vi "Process.vi"(8 "error in":errorcluster, 11 "Logger.Error":refnum<class "Logger.Error.lvclass">) -> (0 "error out":errorcluster, 3 "Logger.Error out":refnum<class "Logger.Error.lvclass">)   [LabVIEW 2019, in "Logger.Error.lvlib" / "Logger.Error.lvclass"]
doc: "---------------------------------------------------------------\nJKI State Machine Objects™\nhttp://jki.net/state-machine-objects/\nCopyright (C) 2005-2015, JKI <info@jki.net>\nALL RIGHTS RESERVED"
uses:
  Logger.Error.lvclass
  C:/Program Files (x86)/National Instruments/LabVIEW 2019/vi.lib/JKI/JKI SMO/smo.lvlibp/SMO/SMO.lvclass
  Logger.Error.lvclass/Logger.Error.ctl
  <vilib>/Utility/file.llb/Write Delimited Spreadsheet (string).vi
  <userlib>/LevyLab/Logger/Logger/Logger.lvclass
  <vilib>/JKI/JKI SMO/smo.lvlibp/SMO/SMO.lvclass
  <userlib>/LevyLab/Debug/Debug.lvlib
panel:
  out "Status":string
  out "State History":string
  # "error Logger"
  # "For instructions on how to use the JKI State Machine Objects, examples and video tutorials, visit:\nhttp://jki.net/state-machine-objects/\n\nJKI State Machine Objects™\nhttp://jki.net/state-machine-objects/\nCopyright (C) 2005-2015, JKI <info@jki.net>\nALL RIGHTS RESERVED"
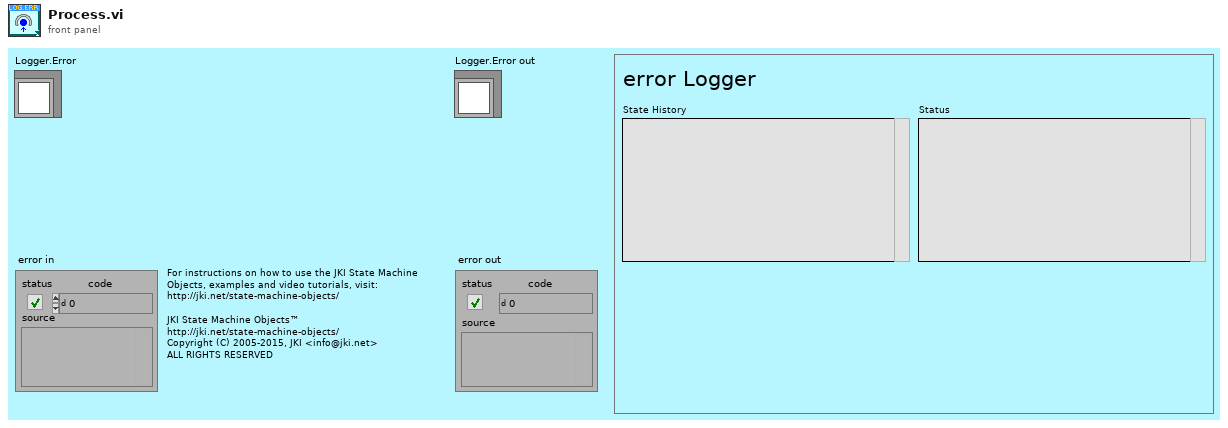
[diagram p1: front panel]
types:
  T1 = enum32{"invalid app kind", "Development System", "Run Time System", "Student Edition", "Embedded LabVIEW", "Evaluation", "Custom"}
  T2 = enum32{"Invalid", "Standard", "Closed", "Hidden", "Minimized", "Maximized"}
  T3 = cluster{"Core":cluster{"Current VI Reference":refnum<vi>, "Close Panel on Exit?":bool, "Last Error":cluster{"error":errorcluster, "previous state":string, "remaining states":string}, "Shutdown?":bool}, "SelfRef":refnum<class "Logger.Error.lvclass">, "path":path, "SMOs":refnum<class "SMO.lvclass">[], "error to log":errorcluster}
  T4 = cluster{"Current VI Reference":refnum<vi>, "Close Panel on Exit?":bool, "Last Error":cluster{"error":errorcluster, "previous state":string, "remaining states":string}, "Shutdown?":bool}
  T5 = typedef "Debug.lvlib/Attribute.Debug.lvclass/DebugBehavior.ctl" = enum16{"Normal", "Debug"}
  T6 = typedef "smo.lvlibp/SMO.lvclass/Protected Events.ctl" = cluster{"StopProcesses":refnum<user-event>, "AbortProcesses":refnum<user-event>, "Config Changed":refnum<user-event>, "Dependency":refnum<user-event>}
  T7 = typedef "smo.lvlibp/SMO.lvclass/Public Events.ctl" = cluster{"Error":refnum<user-event>, "State":refnum<user-event>, "Reserve State":refnum<user-event>}
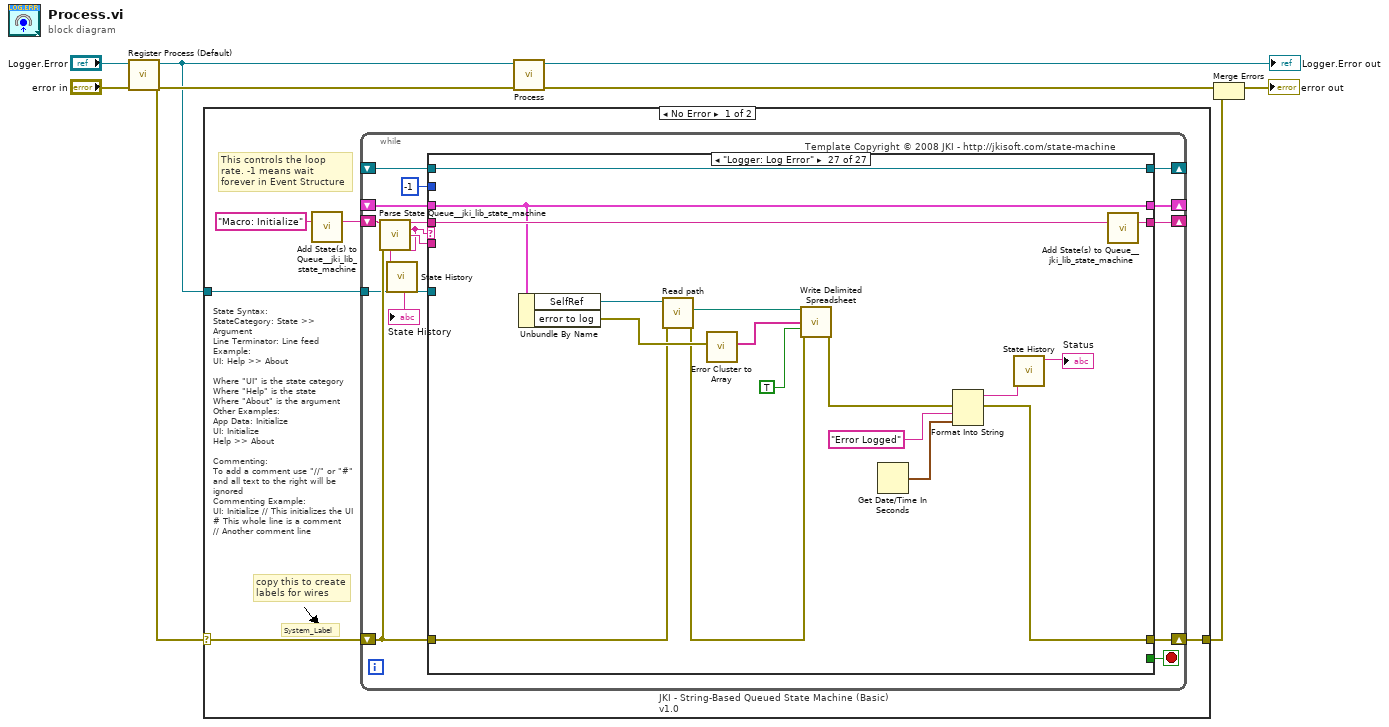
[diagram p0: block diagram]
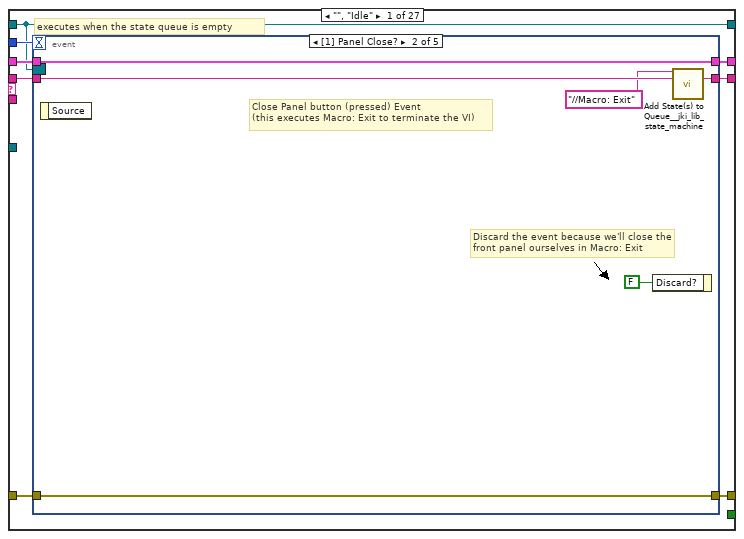
[diagram p2: hidden frame]
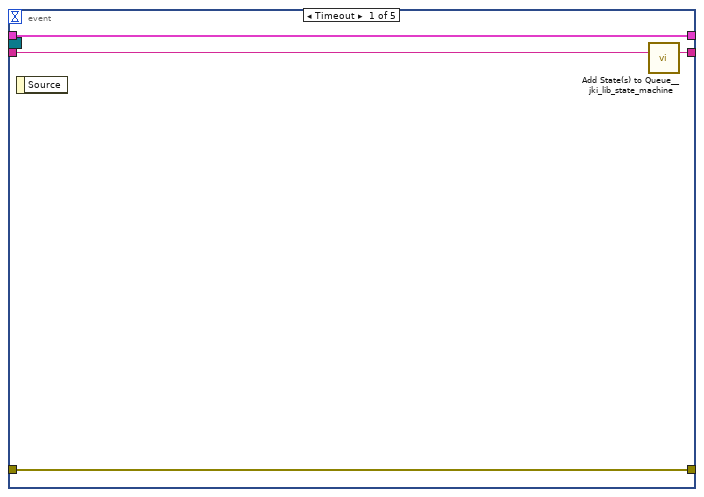
[diagram p3: hidden frame]
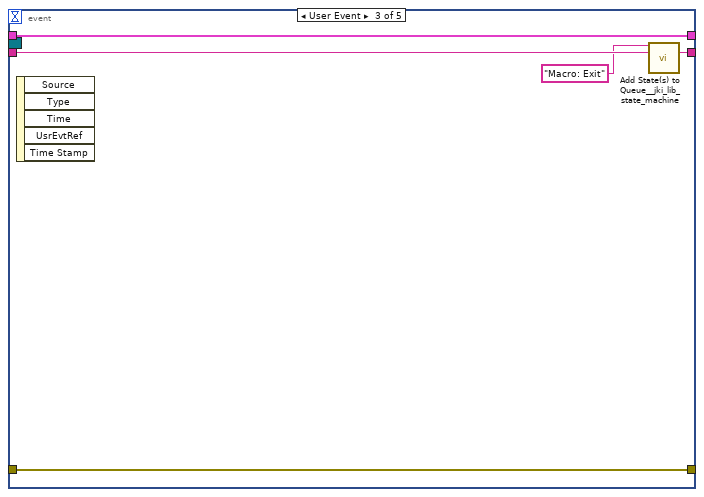
[diagram p4: hidden frame]
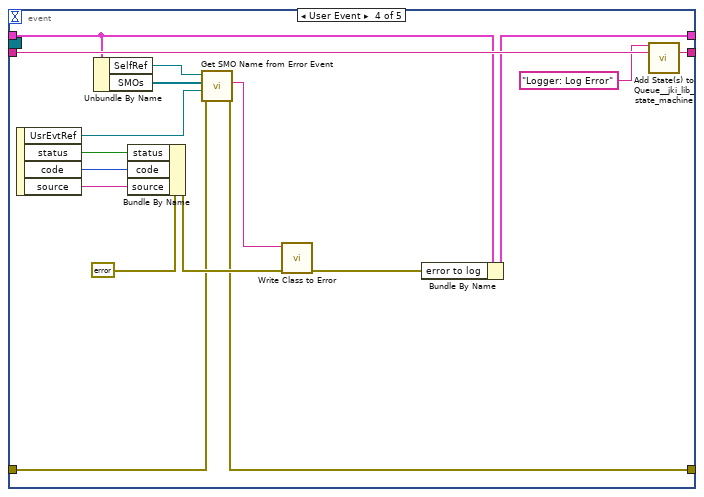
[diagram p5: hidden frame]
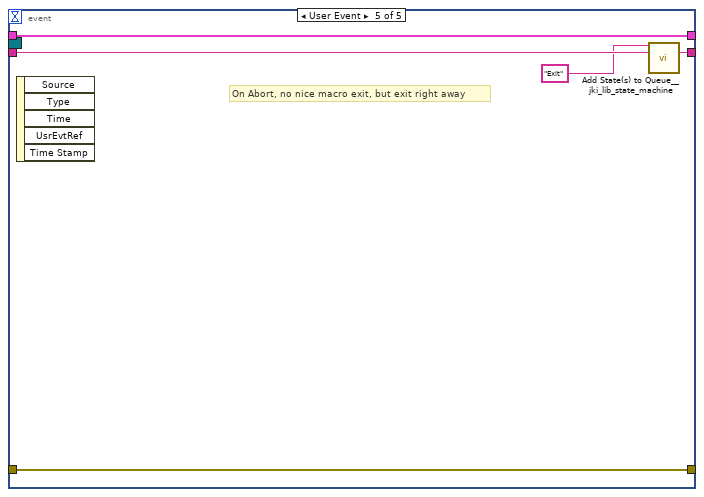
[diagram p6: hidden frame]
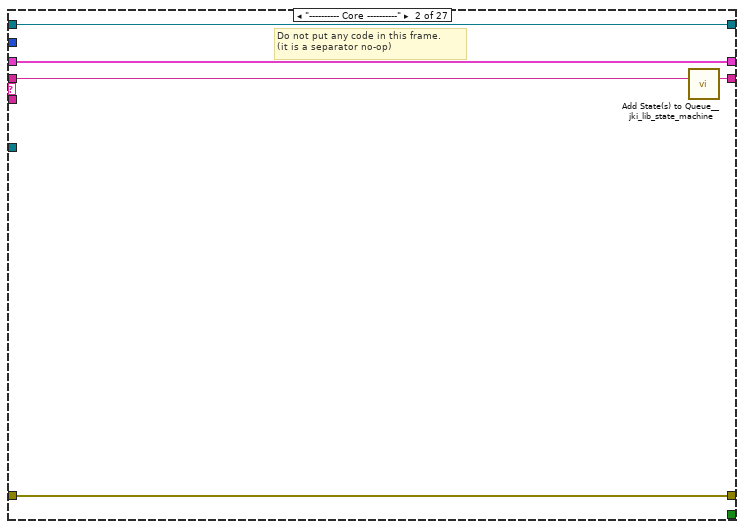
[diagram p7: hidden frame]
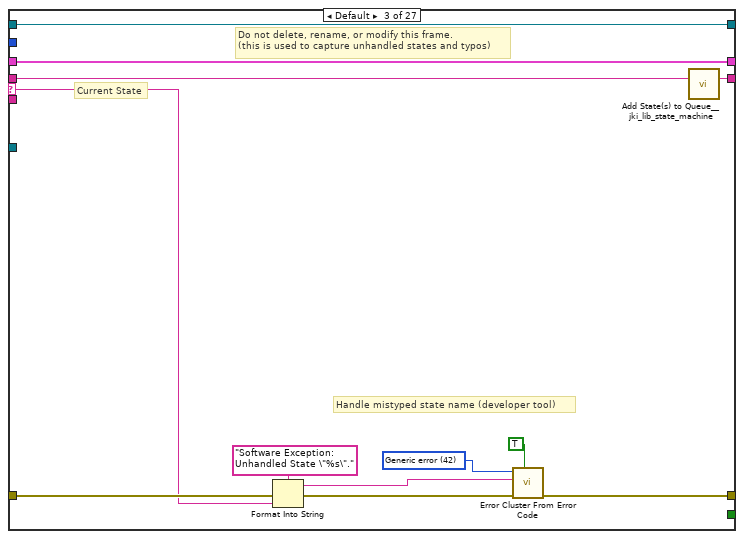
[diagram p8: hidden frame]
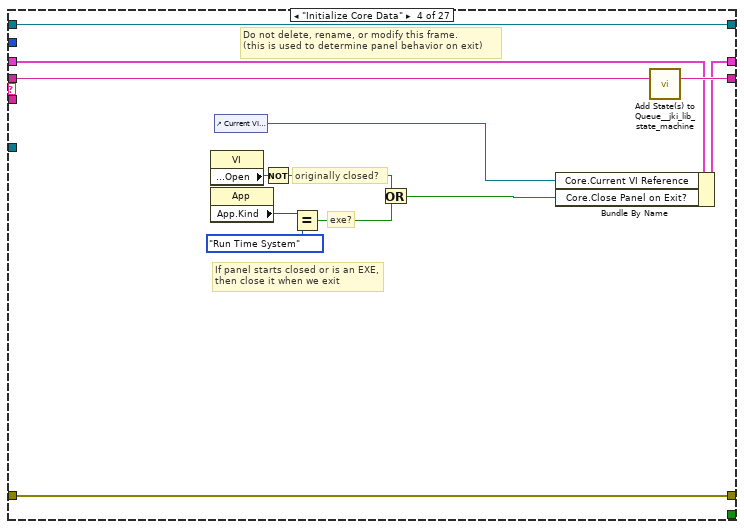
[diagram p9: hidden frame]
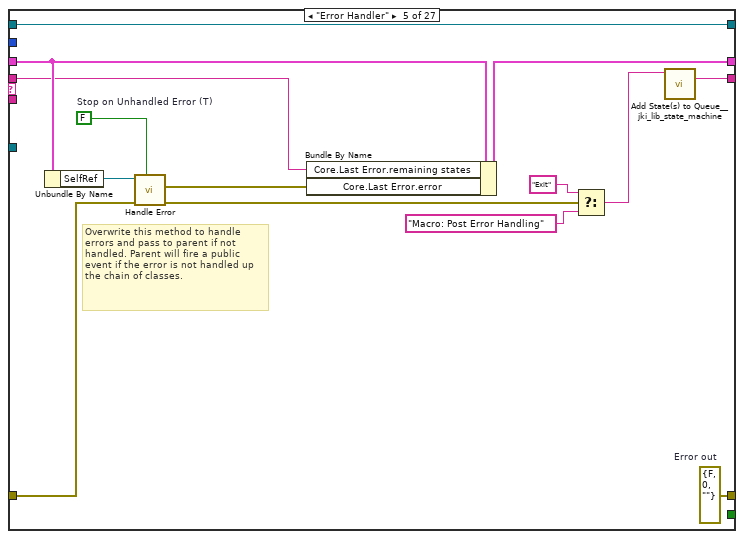
[diagram p10: hidden frame]
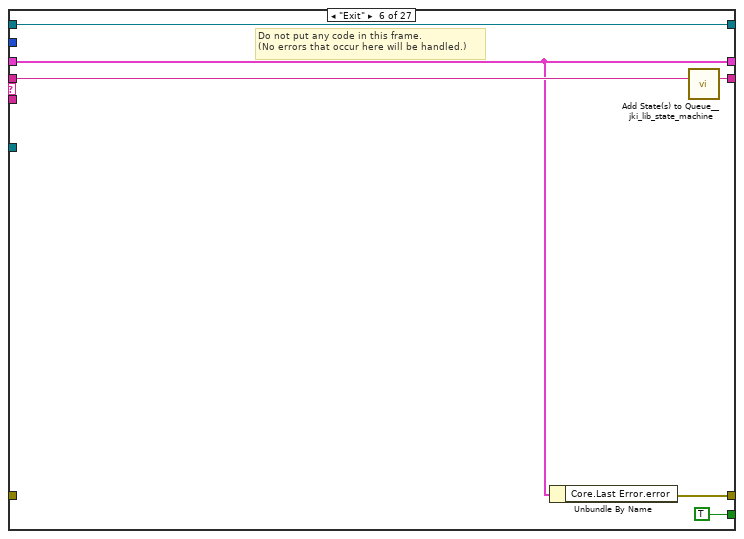
[diagram p11: hidden frame]
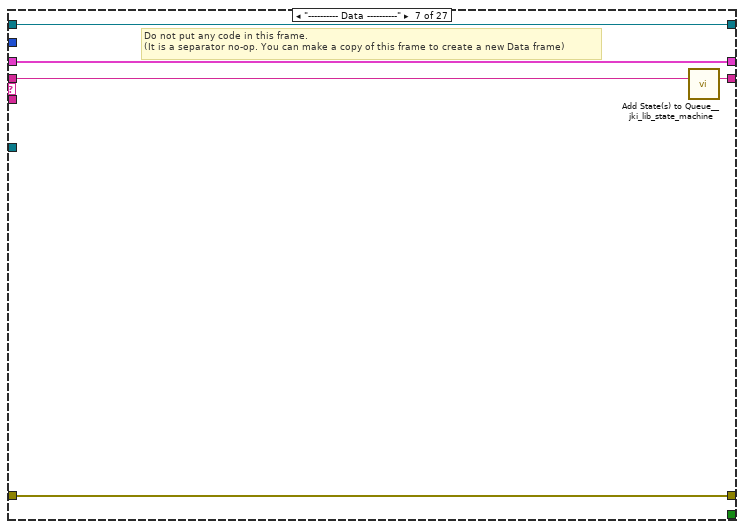
[diagram p12: hidden frame]
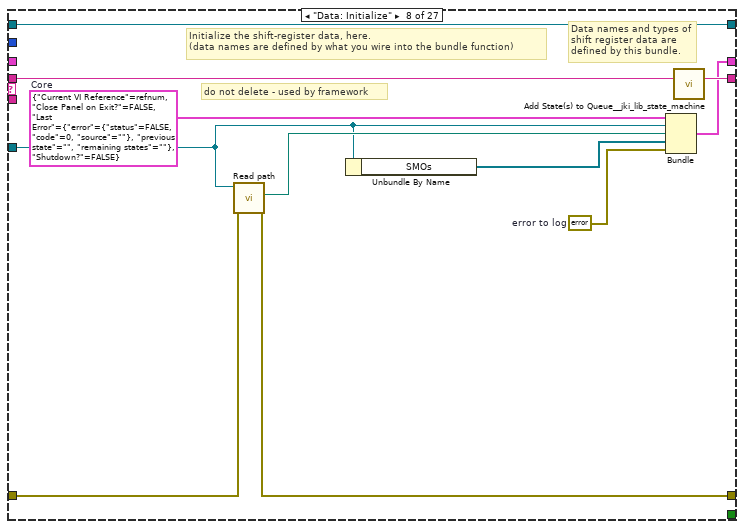
[diagram p13: hidden frame]
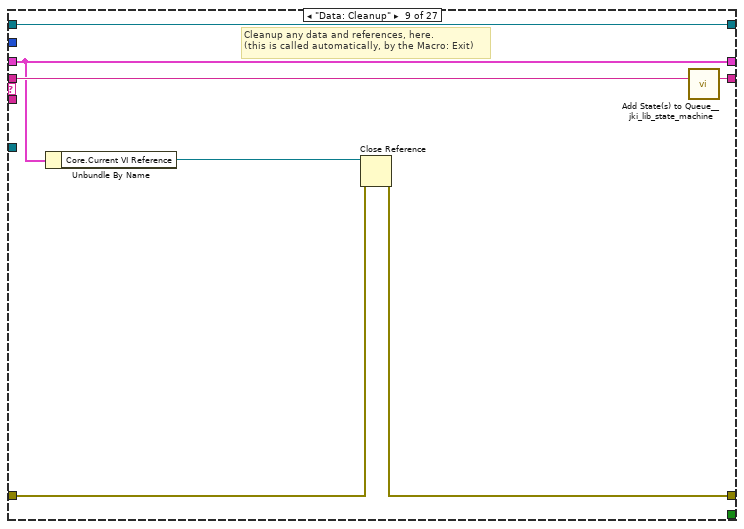
[diagram p14: hidden frame]
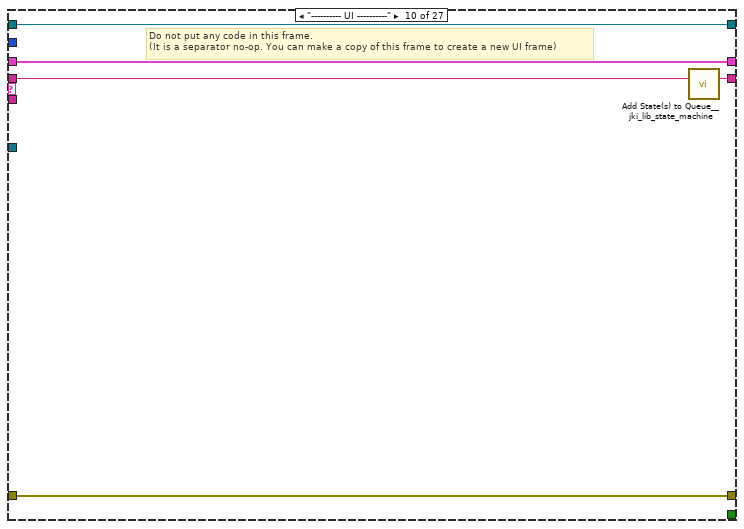
[diagram p15: hidden frame]
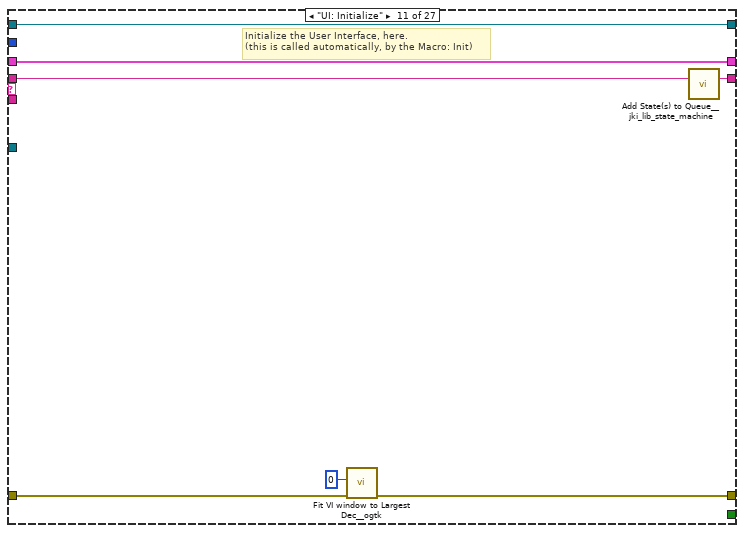
[diagram p16: hidden frame]
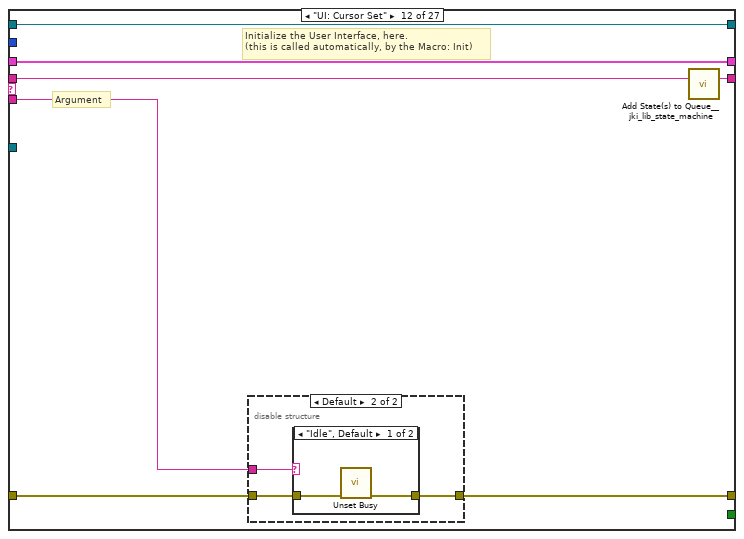
[diagram p17: hidden frame]
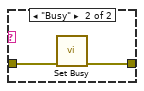
[diagram p19: hidden frame]
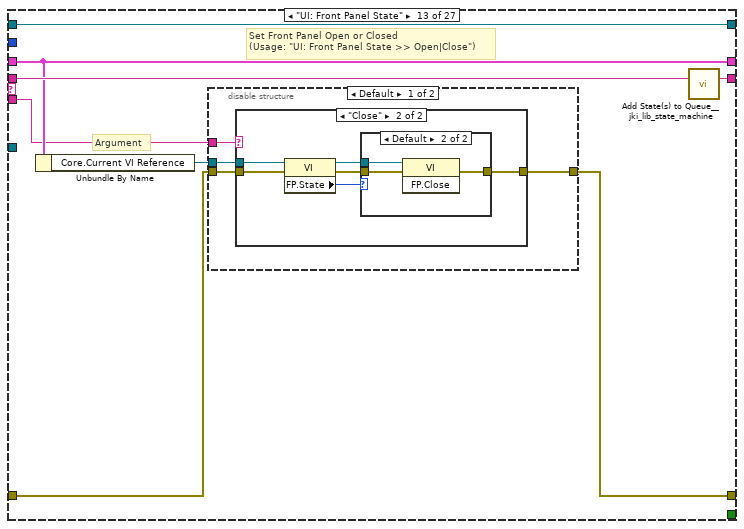
[diagram p20: hidden frame]
diagram:
  n1 = call <vilib>:"Register Process (Default).vi"("error in (no error)"="error in", "SMO"="Logger.Error") -> ("error out"=w5:errorcluster, "SelfRef"=w4:refnum<class "Logger.Error.lvclass">)  [unwired: 8 in]
  n2 = case shown="No Error" w5 {
    selector: w5 -> [w10 w365]
    tunnel: w4 -> [w11 _]
    tunnel: [w9 w365] -> w1
    frame No Error {
      # "State Syntax:\nStateCategory: State >> Argument\nLine Terminator: Line feed\nExample:\nUI: Help >> About\n\nWhere \"UI\" is the state category\nWhere \"Help\" is the state\nWhere \"About\" is the argument\nOther Examples:\nApp Data: Initialize\nUI: Initialize\nHelp >> About\n\nCommenting:\nTo add a comment use \"//\" or \"#\" and all text to the right will be ignored\nCommenting Example:\nUI: Initialize // This initializes the UI\n# This whole line is a comment\n// Another comment line"
      # "copy this to create labels for wires"
      # "This controls the loop rate. -1 means wait forever in Event Structure"
      # "System_Label"
      n3 = call <vilib>:"Add State(s) to Queue__jki_lib_state_machine.vi"("State(s) in (\"\")"="Macro: Initialize") -> ("States Out"=w13:string)  [unwired: 14 in]
      n4 = while "JKI - String-Based Queued State Machine (Basic) v1.0" {
        shift-right: [w22] -> _
        shift-left: _ -> [w14]
        shift-right: [w25] -> w9
        shift-left: w10 -> [w20]
        shift-right: [w24] -> _
        shift-left: w13 -> [w26]
        tunnel: w11 -> [w19]
        shift-right: [w18] -> _
        shift-left: _ -> [w17]
        stop <- w23 stop-if-true
        # "Template Copyright © 2008 JKI - http://jkisoft.com/state-machine"
        n5 = call <vilib>:"Parse State Queue__jki_lib_state_machine.vi"("State Queue"=w26, "Error In (no error)"=w20) -> ("Remaining States"=w28:string, "Current State"=w15:string, "Arguments"=w27:string)  [unwired: 11 in]
        n6 = call <userlib>:"State History.vi"("Current State"=w15) -> ("History"=→"State History":string)  [unwired: 10 in]
        n7 = case shown="\"Logger: Log Error\"" w15 {
          selector: w15 -> [_ _ w80 _ _ _ _ _ _ _ _ _ _ _ _ _ _ _ _ _ _ _ _ _ _ _ _]
          tunnel: w28 -> [w36 w78 w84 w103 w106 w123 w128 w139 w146 w151 w158 w165 w181 w213 w224 w239 w256 w277 w282 w293 w298 w315 w326 w331 w340 w347 w364]
          tunnel: w27 -> [_ _ _ _ _ _ _ _ _ _ _ w159 w175 _ _ _ _ _ _ _ _ _ _ _ _ _ _]
          tunnel: [w33 w76 w86 w100 w113 w118 w126 w131 w142 w149 w153 w160 w178 w211 w215 w226 w254 w275 w280 w284 w296 w311 w322 w327 w336 w341 w349] -> w25
          tunnel: w20 -> [w32 w76 w85 w100 w114 _ w126 w132 w143 w149 w152 w161 w179 w211 w215 w225 w254 w275 w280 w285 w296 w302 w322 w327 w337 w342 w354]
          tunnel: [w35 w77 w83 w102 w117 w122 w127 w138 w145 w150 w157 w164 w180 w212 w223 w238 w255 w276 w281 w292 w297 w314 w325 w330 w339 w346 w363] -> w24
          tunnel: [_ _ _ _ _ TRUE _ _ _ _ _ _ _ _ _ _ _ _ _ _ _ _ _ _ _ _ _] -> w23
          tunnel: [w31 w75 w82 w101 w111 w119 w125 w137 w141 w148 w156 w163 w177 w210 w217 w229 w246 w262 w279 w290 w295 w305 w324 w329 w333 w344 w361] -> w22
          tunnel: -1 ("Timeout") -> [w30 _ _ _ _ _ _ _ _ _ _ _ _ _ _ _ _ _ _ _ _ _ _ _ _ _ _]
          tunnel: w19 -> [_ _ _ _ _ _ _ w130 _ _ _ _ _ _ _ _ _ _ _ _ _ _ _ _ _ _ _]
          tunnel: [w29 w74 w79 w91 w116 w120 w124 w136 w140 w147 w155 w162 w174 w209 w222 w237 w253 w270 w278 w291 w294 w313 w323 w328 w338 w345 w362] -> w18
          tunnel: w17 -> [w29 w74 w79 w91 w116 w120 w124 w136 w140 w147 w155 w162 w174 w209 w222 w237 w253 w270 w278 w291 w294 _ w323 w328 w338 w345 w362]
          tunnel: w14 -> [w34 w75 w82 w94 w112 w119 w125 _ w141 w148 w156 w163 w177 w210 w217 w228 w245 w261 w279 w290 w295 w306 w324 w329 w332 w344 w361]
          frame "", "Idle" {
            # "executes when the state queue is empty"
            n8 = event shown="[1] Panel Close?" {
              selector: w29 -> [_ _ _ _ _]
              dyn-events: _ -> [_ _ _ _ _]
              timeout: w30 -> [_ _ _ _ _]
              tunnel: w36 -> [w40 w46 w51 w68 w73]
              tunnel: [w39 w45 w50 w67 w72] -> w35
              tunnel: w34 -> [w38 w43 w48 w55 w70]
              tunnel: [w37 w44 w49 w57 w71] -> w33
              tunnel: w32 -> [w37 w44 w49 w58 w71]
              tunnel: [w38 w43 w48 w56 w70] -> w31
              event Timeout {
                n9 = event-data() -> ()  [unwired: 1 in, 1 out]
                n10 = call <vilib>:"Add State(s) to Queue__jki_lib_state_machine.vi"("State(s) in (\"\")"=w40) -> ("States Out"=w39:string)  [unwired: 14 in]
              }
              event Panel Close? {
                # "Discard the event because we'll close the front panel ourselves in Macro: Exit"
                # "Close Panel button (pressed) Event\n(this executes Macro: Exit to terminate the VI)"
                n11 = event-data() -> ()  [unwired: 1 in, 1 out]
                n12 = event-data("Discard?"=FALSE) -> ()  [unwired: 1 in, 1 out]
                n13 = call <vilib>:"Add State(s) to Queue__jki_lib_state_machine.vi"("State(s) in Front (\"\")"="//Macro: Exit", "State(s) in (\"\")"=w46) -> ("States Out"=w45:string)  [unwired: 13 in]
              }
              event User Event {
                n14 = event-data() -> ()  [unwired: 1 in, 5 out]
                n15 = call <vilib>:"Add State(s) to Queue__jki_lib_state_machine.vi"("State(s) in Front (\"\")"="Macro: Exit", "State(s) in (\"\")"=w51) -> ("States Out"=w50:string)  [unwired: 13 in]
              }
              event User Event {
                n16 = event-data() -> ("UsrEvtRef"=w62:refnum<user-event>, "status"=w66:bool, "code"=w65:i32, "source"=w64:string)  [unwired: 1 in]
                n17 = Unbundle By Name(w55) -> ("SelfRef"=w52:refnum<class "Logger.Error.lvclass">, "SMOs"=w63:refnum<class "SMO.lvclass">[])
                n18 = Bundle By Name(cluster=errorcluster {"status"=FALSE, "code"=0, "source"=""} ("error in (no error)"), "status"=w66, "code"=w65, "source"=w64) -> (w60:errorcluster)
                n19 = call "Get SMO Name from Error Event.vi"("error in (no error)"=w58, "Error"=w62, "SMOs"=w63, "Logger.Error"=w52) -> ("error out"=w57:errorcluster, "class:SMO name"=w61:string)  [unwired: 5 in, 1 out]
                n20 = call "Write Class to Error.vi"("Error in"=w60, "Calling Class"=w61) -> ("Error out"=w54:errorcluster)  [unwired: 9 in]
                n21 = Bundle By Name(cluster=w55, "error to log"=w54) -> (w56:T3)
                n22 = call <vilib>:"Add State(s) to Queue__jki_lib_state_machine.vi"("State(s) in Front (\"\")"="Logger: Log Error" ("State(s) in Front (\"\")"), "State(s) in (\"\")"=w68) -> ("States Out"=w67:string)  [unwired: 13 in]
              }
              event User Event {
                # "On Abort, no nice macro exit, but exit right away"
                n23 = event-data() -> ()  [unwired: 1 in, 5 out]
                n24 = call <vilib>:"Add State(s) to Queue__jki_lib_state_machine.vi"("State(s) in Front (\"\")"="Exit", "State(s) in (\"\")"=w73) -> ("States Out"=w72:string)  [unwired: 13 in]
              }
            }
          }
          frame "---------- Core ----------" {
            # "Do not put any code in this frame.\n(it is a separator no-op)"
            n25 = call <vilib>:"Add State(s) to Queue__jki_lib_state_machine.vi"("State(s) in (\"\")"=w78) -> ("States Out"=w77:string)  [unwired: 14 in]
          }
          frame Default {
            w89 = 42 items=["No error", "Argument error", "Memory is full", "Out of zone", "End of file", "File already open", "Generic file I/O error", "File not found", "File permission error", "Disk is full", "Duplicate path", "Too many files open", "System feature not enabled", "Resource file not found", "Cannot add resource", "Resource not found", "Image not found", "Image memory error", "Pen does not exist", "Config type invalid", "Config token not found", "Config parse error", "Config memory error", "Bad external code format", "Bad external code offset", "External code not present", "Null window", "Destroy window error", "Null menu", "Print aborted", "Bad print record", "Print driver error", "Windows error during printing", "Memory error during printing", "Print dialog error", "Generic print error", "Invalid device refnum", "Device not found", "Device parameter error", "Device unit error", "Cannot open device", "Device call aborted", "Generic error", "Cancelled by user", "Object ID too low", "Object ID too high", "Object not in heap", "Unknown heap", "Unknown object (invalid DefProc)", "Unknown object (DefProc not in table)", "Message out of range", "Invalid (null) method", "Unknown message", "Manager call not supported", "Bad address", "Network operation in progress", "Network operation timed out", "Connection is busy", "Network attribute not supported", "Network error", "Address in use", "System out of memory", "Connection aborted", "Connection refused", "Not connected", "Already connected", "Connection closed", "Initialization error (interapplication manager)", "Bad occurrence", "Wait on unbound occurrence handler", "Occurrence queue overflow", "Datalog type conflict", "Unused", "Unrecognized type (interapplication manager)", "Memory corrupt", "Failed to make temporary DLL", "Old CIN version", "Drag socket not found", "Failed to load drop-object", "Failed to register OLE object", "Failed to release OLE object", "Format specifier type mismatch", "Unknown format specifier", "Too few format specifiers", "Too many format specifiers", "Scan failed", "Newer CIN version", "Error converting to variant", "Runtime menu error", "Password tampered", "Variant attribute not found", "Incompatible variant data type", "Event data is not available", "Event Store is not present", "Occurrence is not found", "Event Queue is not created", "Event info is not available", "Refnum passed is NULL", "Error retrieving Class GUID", "Error retrieving CoClass GUID", "Error retrieving TypeLib GUID.", "Bad built application magic bytes.", "Specific driver is different from the specific driver associated with the Logical Name.", "There is no session opened to the class driver.", "Max Error", "MAX - Error with config objects", "MAX - Error loading configuration", "MAX - Group not supported"]
            # "Current State"
            # "Do not delete, rename, or modify this frame.\n(this is used to capture unhandled states and typos)"
            # "Handle mistyped state name (developer tool)"
            n26 = Format Into String(format string="Software Exception: Unhandled State \"%s\"." ("message"), error in=w85, w80) -> (resulting string=w88:string, error out=w87:errorcluster)  [unwired: 1 in]
            n27 = call <vilib>:"Error Cluster From Error Code.vi"("show call chain? (False)"=TRUE, "error in (no error)"=w87, "error message (\"\")"=w88, "error code (0)"=w89) -> ("error out"=w86:errorcluster)  [unwired: 5 in]
            n28 = call <vilib>:"Add State(s) to Queue__jki_lib_state_machine.vi"("State(s) in (\"\")"=w84) -> ("States Out"=w83:string)  [unwired: 14 in]
          }
          frame "Initialize Core Data" {
            # "Do not delete, rename, or modify this frame.\n(this is used to determine panel behavior on exit)"
            # "originally closed?"
            # "exe?"
            # "If panel starts closed or is an EXE, then close it when we exit"
            n29 = property class="VI"() -> ("Front Panel.Open"=w99:bool)  [unwired: 2 in, 2 out]
            n30 = property class="App"() -> ("App.Kind"=w98:T1)  [unwired: 2 in, 2 out]
            n31 = control-ref of="Current VI Reference"() -> (w92:refnum<vi>)
            n32 = Not(x=w99) -> (.not. x?=w96:bool)
            n33 = Equal?(x=w98, y=T1."Run Time System" ("Application:Kind")) -> (x = y?=w95:bool)
            n34 = Or(x=w96, y=w95) -> (x .or. y?=w93:bool)
            n35 = Bundle By Name(cluster=w94, "Core.Current VI Reference"=w92, "Core.Close Panel on Exit?"=w93) -> (w101:T3)
            n36 = call <vilib>:"Add State(s) to Queue__jki_lib_state_machine.vi"("State(s) in (\"\")"=w103) -> ("States Out"=w102:string)  [unwired: 14 in]
          }
          frame "Error Handler" {
            w107 = FALSE  # Stop on Unhandled Error (T)
            w113 = errorcluster {"status"=FALSE, "code"=0, "source"=""}  # Error out
            # "Overwrite this method to handle errors and pass to parent if not handled. Parent will fire a public event if the error is not handled up the chain of classes."
            n37 = Unbundle By Name(w112) -> ("SelfRef"=w115:refnum<class "Logger.Error.lvclass">)
            n38 = call-dynamic "Handle Error.vi"("Stop on Unhandled Error (T)"=w107, "error in"=w114, "SMO"=w115) -> ("handling error"=w108:errorcluster, "Unhandled error"=w104:errorcluster)  [unwired: 6 in, 1 out]
            n39 = Bundle By Name(cluster=w112, "Core.Last Error.remaining states"=w106, "Core.Last Error.error"=w104) -> (w111:T3)
            n40 = Select(t="Exit", s=w108, f="Macro: Post Error Handling") -> (s? t:f=w110:string)
            n41 = call <vilib>:"Add State(s) to Queue__jki_lib_state_machine.vi"("State(s) in Front (\"\")"=w110) -> ("States Out"=w117:string)  [unwired: 14 in]
          }
          frame "Exit" {
            # "Do not put any code in this frame.\n(No errors that occur here will be handled.)"
            n42 = Unbundle By Name(w119) -> ("Core.Last Error.error"=w118:errorcluster)
            n43 = call <vilib>:"Add State(s) to Queue__jki_lib_state_machine.vi"("State(s) in (\"\")"=w123) -> ("States Out"=w122:string)  [unwired: 14 in]
          }
          frame "---------- Data ----------" {
            # "Do not put any code in this frame.\n(It is a separator no-op. You can make a copy of this frame to create a new Data frame)"
            n44 = call <vilib>:"Add State(s) to Queue__jki_lib_state_machine.vi"("State(s) in (\"\")"=w128) -> ("States Out"=w127:string)  [unwired: 14 in]
          }
          frame "Data: Initialize" {
            w133 = errorcluster {"status"=FALSE, "code"=0, "source"=""}  # error to log
            w135 = T4 {"Current VI Reference"=refnum, "Close Panel on Exit?"=FALSE, "Last Error"={"error"={"status"=FALSE, "code"=0, "source"=""}, "previous state"="", "remaining states"=""}, "Shutdown?"=FALSE}  # Core
            # "do not delete - used by framework"
            # "Data names and types of shift register data are defined by this bundle."
            # "Initialize the shift-register data, here.\n(data names are defined by what you wire into the bundle function)"
            n45 = call-dynamic "Read path.vi"("error in (no error)"=w132, "Logger in"=w130) -> ("error out"=w131:errorcluster, "path"=w134:path)  [unwired: 7 in, 1 out]
            n46 = Unbundle By Name(w130) -> ("SMOs"=w129:refnum<class "SMO.lvclass">[])
            n47 = Bundle("Core"=w135, "SelfRef"=w130, "path"=w134, "SMOs"=w129, "error to log"=w133) -> (w137:T3)  [unwired: 1 in]
            n48 = call <vilib>:"Add State(s) to Queue__jki_lib_state_machine.vi"("State(s) in (\"\")"=w139) -> ("States Out"=w138:string)  [unwired: 14 in]
          }
          frame "Data: Cleanup" {
            # "Cleanup any data and references, here.\n(this is called automatically, by the Macro: Exit)"
            n49 = Unbundle By Name(w141) -> ("Core.Current VI Reference"=w144:refnum<vi>)
            n50 = Close Reference(reference=w144, error in (no error)=w143) -> (error out=w142:errorcluster)
            n51 = call <vilib>:"Add State(s) to Queue__jki_lib_state_machine.vi"("State(s) in (\"\")"=w146) -> ("States Out"=w145:string)  [unwired: 14 in]
          }
          frame "---------- UI ----------" {
            # "Do not put any code in this frame.\n(It is a separator no-op. You can make a copy of this frame to create a new UI frame)"
            n52 = call <vilib>:"Add State(s) to Queue__jki_lib_state_machine.vi"("State(s) in (\"\")"=w151) -> ("States Out"=w150:string)  [unwired: 14 in]
          }
          frame "UI: Initialize" {
            # "Initialize the User Interface, here.\n(this is called automatically, by the Macro: Init)"
            n53 = call <userlib>:"Fit VI window to Largest Dec__ogtk.vi"("error in (no error)"=w152, "border spacing (2 px)"=0) -> ("error out"=w153:errorcluster)  [unwired: 4 in, 1 out]
            n54 = call <vilib>:"Add State(s) to Queue__jki_lib_state_machine.vi"("State(s) in (\"\")"=w158) -> ("States Out"=w157:string)  [unwired: 14 in]
          }
          frame "UI: Cursor Set" {
            # "Argument"
            # "Initialize the User Interface, here.\n(this is called automatically, by the Macro: Init)"
            n55 = disable-structure shown="Default" {
              disable-tunnel: w161 -> [w166 w169]
              disable-tunnel: [w166 w168] -> w160
              disable-tunnel: w159 -> [_ w167]
              frame condition #0 {
              }
              frame condition #1 (active) {
                n56 = case shown="\"Idle\", Default" w167 {
                  tunnel: w169 -> [w171 w173]
                  tunnel: [w170 w172] -> w168
                  frame "Idle", Default {
                    n57 = call <vilib>:"Unset Busy.vi"("error in (no error)"=w171) -> ("error out"=w170:errorcluster)  [unwired: 10 in]
                  }
                  frame "Busy" {
                    n58 = call <vilib>:"Set Busy.vi"("error in (no error)"=w173) -> ("error out"=w172:errorcluster)  [unwired: 9 in, 1 out]
                  }
                }
              }
            }
            n59 = call <vilib>:"Add State(s) to Queue__jki_lib_state_machine.vi"("State(s) in (\"\")"=w165) -> ("States Out"=w164:string)  [unwired: 14 in]
          }
          frame "UI: Front Panel State" {
            # "Argument"
            # "Set Front Panel Open or Closed\n(Usage: \"UI: Front Panel State >> Open|Close\")"
            n60 = Unbundle By Name(w177) -> ("Core.Current VI Reference"=w176:refnum<vi>)
            n61 = disable-structure shown="Default" {
              disable-tunnel: w179 -> [w185 w208]
              disable-tunnel: [w184 w208] -> w178
              disable-tunnel: w176 -> [w183 _]
              disable-tunnel: w175 -> [w182 _]
              frame condition #0 (active) {
                n62 = case shown="\"Close\"" w182 {
                  tunnel: w185 -> [w189 w202]
                  tunnel: [w191 w203] -> w184
                  tunnel: w183 -> [w190 w200]
                  frame "Open", Default {
                    n63 = property class="VI"(reference=w190, error in=w189) -> (reference out=w187:refnum<vi>, error out=w188:errorcluster, "FP.State"=w186:T2)
                    n64 = case shown="\"Closed\"" w186 {
                      tunnel: [w194 w197] -> w191
                      tunnel: w188 -> [w193 w197]
                      tunnel: w187 -> [w192 _]
                      frame "Closed" {
                        n65 = invoke class="VI" method="FP.Open"(reference=w192, error in=w193, "Activate"=TRUE, "State"=T2."Standard") -> (error out=w194:errorcluster)  [unwired: 1 in, 4 out]
                      }
                      frame Default {
                      }
                    }
                  }
                  frame "Close" {
                    n66 = property class="VI"(reference=w200, error in=w202) -> (reference out=w199:refnum<vi>, error out=w201:errorcluster, "FP.State"=w198:T2)
                    n67 = case shown="Default" w198 {
                      tunnel: [w204 w207] -> w203
                      tunnel: w201 -> [w204 w206]
                      tunnel: w199 -> [_ w205]
                      frame "Invalid", "Closed" {
                      }
                      frame Default {
                        n68 = invoke class="VI" method="FP.Close"(reference=w205, error in=w206) -> (error out=w207:errorcluster)  [unwired: 1 in, 2 out]
                      }
                    }
                  }
                }
              }
              frame condition #1 {
              }
            }
            n69 = call <vilib>:"Add State(s) to Queue__jki_lib_state_machine.vi"("State(s) in (\"\")"=w181) -> ("States Out"=w180:string)  [unwired: 14 in]
          }
          frame "---------- Macro ----------" {
            # "Do not put any code in this frame.\n(It is a separator no-op. You can make a copy of this frame to create a new Macro frame)"
            n70 = call <vilib>:"Add State(s) to Queue__jki_lib_state_machine.vi"("State(s) in (\"\")"=w213) -> ("States Out"=w212:string)  [unwired: 14 in]
          }
          frame "Macro: Initialize" {
            # "Initialization Macro\n(This is called once, when the VI starts)"
            n71 = call <vilib>:"Add State(s) to Queue__jki_lib_state_machine.vi"("State(s) in Front (\"\")"="UI: Initialize", "State(s) in (\"\")"="UI: Front Panel State >> Close\nMacro: Debug\nLogger: Start Error Logger") -> ("States Out"=w216:string)  [unwired: 13 in]
            n72 = call <vilib>:"Add State(s) to Queue__jki_lib_state_machine.vi"("State(s) in Front (\"\")"="Data: Initialize\nInitialize Core Data\nEvents: Register", "State(s) in (\"\")"="Process: Sync", "State(s) at Back (\"\")"=w216) -> ("States Out"=w220:string)  [unwired: 12 in]
            n73 = call <vilib>:"Add State(s) to Queue__jki_lib_state_machine.vi"("State(s) in Front (\"\")"=w220, "State(s) in (\"\")"=w224) -> ("States Out"=w223:string)  [unwired: 13 in]
          }
          frame "Macro: Debug" {
            # "exe?"
            # "If pane is an EXE, then close it when we exit"
            # "Macro: Debug\n(get debug behavior, determine UI and determine shutdown behavior)"
            n74 = Unbundle By Name(w228) -> ("Core.Close Panel on Exit?"=w231:bool, "SelfRef"=w236:refnum<class "Logger.Error.lvclass">)
            n75 = property class="App"() -> ("App.Kind"=w234:T1)  [unwired: 2 in, 2 out]
            n76 = Equal?(x=w234, y=T1."Run Time System" ("Application:Kind")) -> (x = y?=w230:bool)
            n77 = call <userlib>:"Get Debug Mode.vi"("error in (no error)"=w225, "SMO"=w236) -> ("error out"=w226:errorcluster, "Behavior"=w235:T5)  [unwired: 7 in, 1 out]
            n78 = case shown="\"Debug\"" w235 {
              tunnel: [w240 w242] -> w232
              tunnel: w231 -> [w240 _]
              tunnel: w230 -> [_ w244]
              tunnel: [_ "UI: Front Panel State >> Open\nUI: Wait >> 1000"] -> w227
              frame "Normal", Default {
                # "respect core.close"
              }
              frame "Debug" {
                # "keep panel open\nunless exe"
                n79 = Or(x=w244, y=FALSE) -> (x .or. y?=w242:bool)
              }
            }
            n80 = Bundle By Name(cluster=w228, "Core.Close Panel on Exit?"=w232) -> (w229:T3)
            n81 = call <vilib>:"Add State(s) to Queue__jki_lib_state_machine.vi"("State(s) in Front (\"\")"=w227, "State(s) in (\"\")"=w239) -> ("States Out"=w238:string)  [unwired: 13 in]
          }
          frame "Macro: Post Error Handling" {
            # "Clear Last Error?"
            n82 = Unbundle By Name(w245) -> ("Core.Last Error.remaining states"=w248:string, "Core.Shutdown?"=w249:bool)
            n83 = Unbundle By Name(w245) -> ("Core.Last Error.error"=w252:errorcluster)
            n84 = case shown="False" FALSE {
              tunnel: w252 -> [w260 _]
              tunnel: [w260 _] -> w251
              frame False {
              }
              frame True {
              }
            }
            n85 = case shown="False" w249 {
              tunnel: w248 -> [w257 w259]
              tunnel: [w257 w258] -> w247
              frame False {
                # "These are the remaining states (at the moment the error occured). States can be altered according to business logic."
                # "NOT SHUTTING DOWN"
              }
              frame True {
                # "Developer can decide to alter the states but should be aware that during the shutdown process, there are certain states that must be run for the SMO to properly shut itself (and this process) down. As such, one can add states to perform additional clean-ups, but should append the remaining state to be executed."
                # "SHUTTING DOWN"
                n86 = call <vilib>:"Add State(s) to Queue__jki_lib_state_machine.vi"("State(s) in (\"\")"=w259) -> ("States Out"=w258:string)  [unwired: 14 in]
              }
            }
            n87 = Bundle By Name(cluster=w245, "Core.Last Error.error"=w251) -> (w246:T3)
            n88 = call <vilib>:"Add State(s) to Queue__jki_lib_state_machine.vi"("State(s) in Front (\"\")"=w247, "State(s) in (\"\")"=w256) -> ("States Out"=w255:string)  [unwired: 13 in]
          }
          frame "Macro: Exit" {
            # "Exit Macro\n(This is called once, when the VI exits)"
            n89 = Unbundle By Name(w261) -> ("Core.Close Panel on Exit?"=w274:bool)
            n90 = Bundle By Name(cluster=w261, "Core.Shutdown?"=TRUE) -> (w262:T3)
            n91 = Select(t="UI: Front Panel State >> Close", s=w274, f="") -> (s? t:f=w272:string)
            n92 = call <vilib>:"Add State(s) to Queue__jki_lib_state_machine.vi"("State(s) in Front (\"\")"="Logger: Stop Error Logger\nData: Cleanup\nEvents: Unregister", "State(s) in (\"\")"="Process: Sync", "State(s) at Back (\"\")"="Exit") -> ("States Out"=w267:string)  [unwired: 12 in]
            n93 = call <vilib>:"Add State(s) to Queue__jki_lib_state_machine.vi"("State(s) in Front (\"\")"="" ("State(s) in Front (\"\")"), "State(s) in (\"\")"=w272, "State(s) at Back (\"\")"=w267) -> ("States Out"=w271:string)  [unwired: 12 in]
            n94 = call <vilib>:"Add State(s) to Queue__jki_lib_state_machine.vi"("State(s) in Front (\"\")"=w271, "State(s) in (\"\")"=w277) -> ("States Out"=w276:string)  [unwired: 13 in]
          }
          frame "---------- Process ----------" {
            # "Template Separator\n(You can make a copy of, or modify, this frame)"
            n95 = call <vilib>:"Add State(s) to Queue__jki_lib_state_machine.vi"("State(s) in (\"\")"=w282) -> ("States Out"=w281:string)  [unwired: 14 in]
          }
          frame "Process: Sync" {
            n96 = Unbundle By Name(w290) -> ("SelfRef"=w286:refnum<class "Logger.Error.lvclass">)
            n97 = call <vilib>:"WaitOnProcessSync.vi"("error in (no error)"=w285, "SMO"=w286) -> ("error out"=w284:errorcluster, "Don't run?"=w289:bool)  [unwired: 7 in, 1 out]
            n98 = Select(t="Data: Cleanup\nEvents: Unregister\nExit", s=w289, f="") -> (s? t:f=w283:string)
            n99 = call <vilib>:"Add State(s) to Queue__jki_lib_state_machine.vi"("State(s) in Front (\"\")"=w283, "State(s) in (\"\")"=w293) -> ("States Out"=w292:string)  [unwired: 13 in]
          }
          frame "---------- Events ----------" {
            # "Template Separator\n(You can make a copy of, or modify, this frame)"
            n100 = call <vilib>:"Add State(s) to Queue__jki_lib_state_machine.vi"("State(s) in (\"\")"=w298) -> ("States Out"=w297:string)  [unwired: 14 in]
          }
          frame "Events: Register" {
            n101 = Unbundle By Name(w306) -> ("SelfRef"=w312:refnum<class "Logger.Error.lvclass">)
            n102 = call <vilib>:"GetProtectedEvents.vi"("SMO"=w312) -> ("error out"=w310:errorcluster, "SMO Protected Events"=w309:T6, "SMO out"=w308:refnum<class "Logger.Error.lvclass">)  [unwired: 8 in]
            n103 = Unbundle By Name(w308) -> ("SMOs"=w300:refnum<class "SMO.lvclass">[])
            n104 = Build Array (concatenate)(w300, w308) -> (w307:refnum<class "SMO.lvclass">[])
            n105 = for {
              tunnel: w307 -> [w319] mode=indexing
              tunnel: [w318] -> w304 mode=indexing
              tunnel: [w316] -> w303 mode=indexing
              tunnel: [w317] -> w299 mode=indexing
              n106 = call <vilib>:"GetPublicEvents.vi"("SMO"=w319) -> ("error out"=w317:errorcluster, "Public Events"=w320:T7, "SMO out"=w316:refnum<class "SMO.lvclass">)  [unwired: 8 in]
              n107 = Unbundle By Name(w320) -> ("Error"=w318:refnum<user-event>)
            }
            n108 = register-events(w309, w304) -> (reference out=w313:refnum<event-registration>, error out=w301:errorcluster)  [unwired: 2 in]
            n109 = Bundle By Name(cluster=w306, "SMOs"=w303) -> (w305:T3)
            n110 = Merge Errors(w301, w299, w310, w302) -> (w311:errorcluster)
            n111 = call <vilib>:"Add State(s) to Queue__jki_lib_state_machine.vi"("State(s) in (\"\")"=w315) -> ("States Out"=w314:string)  [unwired: 14 in]
          }
          frame "Events: Unregister" {
            n112 = Unregister For Events(event registration refnum=w323, error in=w322) -> (error out=w321:errorcluster)
            n113 = call <vilib>:"Clear Errors.vi"("error in (no error)"=w321) -> ()  [unwired: 5 in, 2 out]
            n114 = call <vilib>:"Add State(s) to Queue__jki_lib_state_machine.vi"("State(s) in (\"\")"=w326) -> ("States Out"=w325:string)  [unwired: 14 in]
          }
          frame "---------- Logger ----------" {
            n115 = call <vilib>:"Add State(s) to Queue__jki_lib_state_machine.vi"("State(s) in (\"\")"=w331) -> ("States Out"=w330:string)  [unwired: 14 in]
          }
          frame "Logger: Start Error Logger" {
            # "will these work with other SMOs?"
            n116 = Unbundle By Name(w332) -> ("SelfRef"=w335:refnum<class "Logger.Error.lvclass">)
            n117 = call-dynamic "Create Logger.vi"("error in (no error)"=w337, "Logger.Error in"=w335) -> ("error out"=w336:errorcluster, "Logger.Error out"=w334:refnum<class "Logger.Error.lvclass">)  [unwired: 8 in]
            n118 = Bundle By Name(cluster=w332, "SelfRef"=w334) -> (w333:T3)
            n119 = call <vilib>:"Add State(s) to Queue__jki_lib_state_machine.vi"("State(s) in (\"\")"=w340) -> ("States Out"=w339:string)  [unwired: 14 in]
          }
          frame "Logger: Stop Error Logger" {
            n120 = Unbundle By Name(w344) -> ("SelfRef"=w343:refnum<class "Logger.Error.lvclass">)
            n121 = call-dynamic "Destroy Logger.vi"("error in (no error)"=w342, "Logger.Error in"=w343) -> ("error out"=w341:errorcluster)  [unwired: 8 in, 1 out]
            n122 = call <vilib>:"Add State(s) to Queue__jki_lib_state_machine.vi"("State(s) in (\"\")"=w347) -> ("States Out"=w346:string)  [unwired: 14 in]
          }
          frame "Logger: Log Error" {
            n123 = Unbundle By Name(w361) -> ("SelfRef"=w357:refnum<class "Logger.Error.lvclass">, "error to log"=w359:errorcluster)
            n124 = call-dynamic "Read path.vi"("error in (no error)"=w354, "Logger in"=w357) -> ("error out"=w355:errorcluster, "path"=w356:path)  [unwired: 7 in, 1 out]
            n125 = call "Error Cluster to Array.vi"("error in (no error)"=w359) -> ("Error Array"=w358:string[])  [unwired: 10 in]
            n126 = call-poly <vilib>:"Write Delimited Spreadsheet.vi"("file path (dialog if empty)"=w356, "1D data"=w358, "append to file? (new file:F)"=TRUE, "error in (no error)"=w355) -> ("error out"=w350:errorcluster)  [unwired: 10 in, 1 out]
            n127 = Get Date/Time In Seconds() -> (seconds since 1Jan1904=w352:timestamp)
            n128 = Format Into String(error in=w350, "Error Logged", w352) -> (resulting string=w351:string, error out=w349:errorcluster)  [unwired: 2 in]
            n129 = call <userlib>:"State History.vi"("Current State"=w351) -> ("History"=→"Status":string)  [unwired: 10 in]
            n130 = call <vilib>:"Add State(s) to Queue__jki_lib_state_machine.vi"("State(s) in (\"\")"=w364) -> ("States Out"=w363:string)  [unwired: 14 in]
          }
        }
      }
    }
    frame Error {
    }
  }
  n131 = call-parent "Process.vi"("error in"=w5, "Logger"=w4) -> ("error out"=w2:errorcluster, "Logger out"=→"Logger.Error out":refnum<class "Logger.Error.lvclass">)  [unwired: 8 in]
  n132 = Merge Errors(w2, w1) -> (→"error out":errorcluster)
